vi "QueryVelocityState.vi"(1 "Destination":T1={"Subsystem Id"=90, "Node Id"=1, "Component Id"=1}, 2 "PresenceVector":u16=2, 3 "Source":T1={"Subsystem Id"=3, "Node Id"=1, "Component Id"=1}) -> (0 "Encoded JAUS Message":string)   [LabVIEW 2009]
uses:
  Support Files/Address.ctl
panel:
  in  "Time Stamp":bool
  in  "Rate RMS":bool
  in  "Yaw Rate":bool
  in  "Pitch Rate":bool
  in  "Roll Rate":bool
  in  "Velocity RMS":bool
  in  "Velocity Z":bool
  in  "Velocity Y":bool
  in  "Velocity X":bool
  in  "Command Code":string="$\u0004"
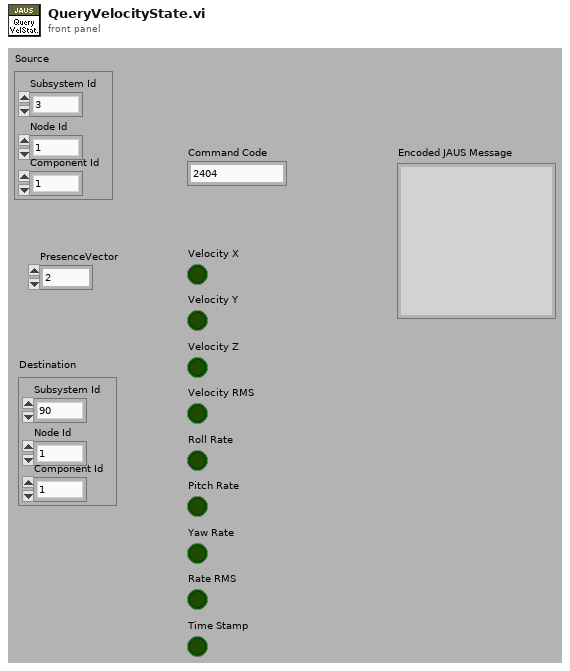
[diagram p1: front panel]
types:
  T1 = typedef "Address.ctl" = cluster{"Subsystem Id":u16, "Node Id":u8, "Component Id":u8}
  T2 = cluster{"unsigned byte array[0]":u8, "unsigned byte array[1]":u8}
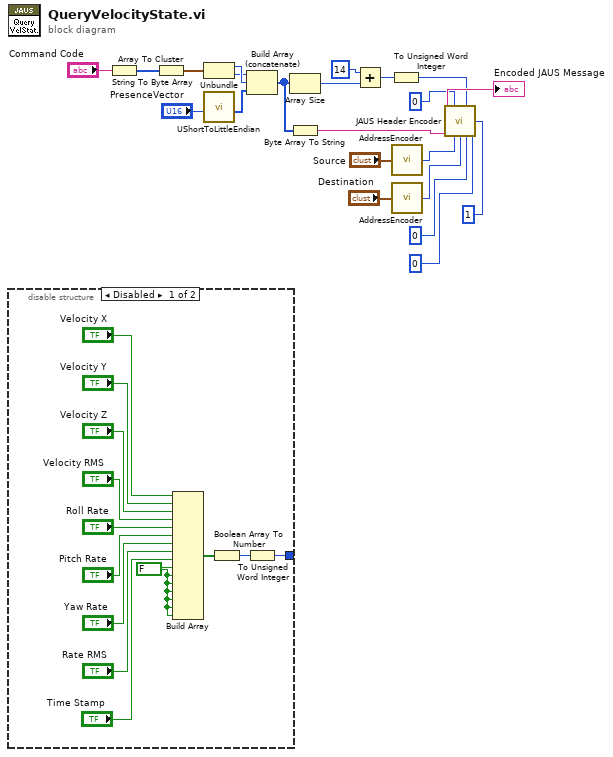
[diagram p0: block diagram]
diagram:
  n1 = disable-structure shown="Disabled" {
    disable-tunnel: [w23 _] -> _
    frame #0 {
      w26 = FALSE
      n2 = Build Array("Velocity X", "Velocity Y", "Velocity Z", "Velocity RMS", "Roll Rate", "Pitch Rate", "Yaw Rate", "Rate RMS", "Time Stamp", w26, w26, w26, w26, w26, w26, w26) -> (w25:bool[])
      n3 = Boolean Array To Number(Boolean array=w25) -> (number=w24:u32)
      n4 = To Unsigned Word Integer(number=w24) -> (unsigned 16bit integer=w23:u16)
    }
    frame #1 {
    }
  }
  n5 = String To Byte Array(string="Command Code") -> (unsigned byte array=w9:u8[])
  n6 = Array To Cluster(array=w9) -> (cluster=w8:T2)
  n7 = Unbundle(w8) -> ("unsigned byte array[0]"=w7:u8, "unsigned byte array[1]"=w6:u8)
  n8 = call "UShortToLittleEndian.vi"("Number"="PresenceVector") -> ("byte array"=w2:u8[])  [unwired: 10 in]
  n9 = Build Array (concatenate)(w6, w7, w2) -> (w13:u8[])
  n10 = Array Size(array=w13) -> (size(s)=w11:i32)
  n11 = Byte Array To String(unsigned byte array=w13) -> (string=w15:string)
  n12 = Add(x=14, y=w11) -> (x+y=w10:i32)
  n13 = To Unsigned Word Integer(number=w10) -> (unsigned 16bit integer=w3:u16)
  n14 = call "AddressEncoder.vi"("Address Cluster"="Source") -> ("Address"=w21:u32)
  n15 = call "AddressEncoder.vi"("Address Cluster"="Destination") -> ("Address"=w20:u32)
  n16 = call "JAUS Header Encoder.vi"("Message Type (0-5)"=u8 0, "Data Size (8-23)"=w3, "Priority(40-41)"=u8 1, "Payload"=w15, "Source ID (80-95)"=w21, "Destination ID (48-79)"=w20, "Data Flags (46-47)"=u8 0, "Ack/Nak (44-45)"=u8 0) -> ("Encoded JAUS Message"=→"Encoded JAUS Message":string)  [unwired: 7 in]
